vi "Is palindrome-number.vi"(8 "error in (no error)":errorcluster, 11 "x":u64) -> (0 "error out":errorcluster, 3 "T = x is a palindrome":bool)   [LabVIEW 2021, in "Numeric Utilities.lvlib"]
uses:
  Numeric Utilities.lvlib
panel:
  out "x (string representation)":string
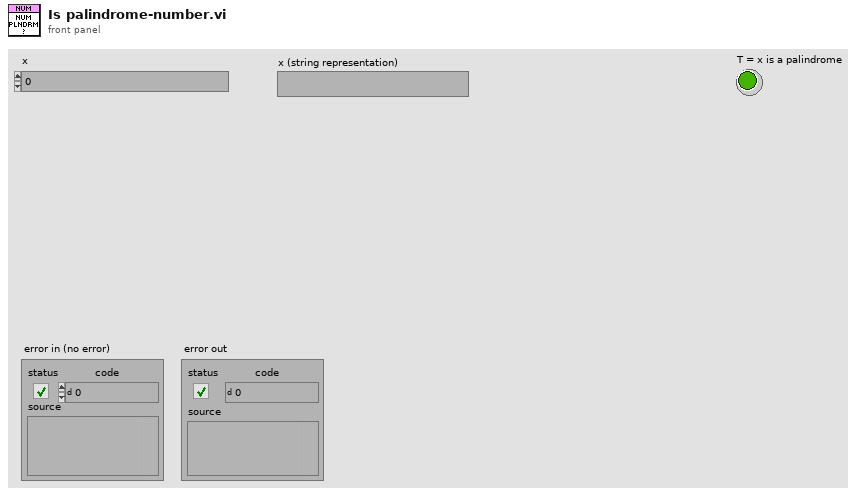
[diagram p1: front panel]
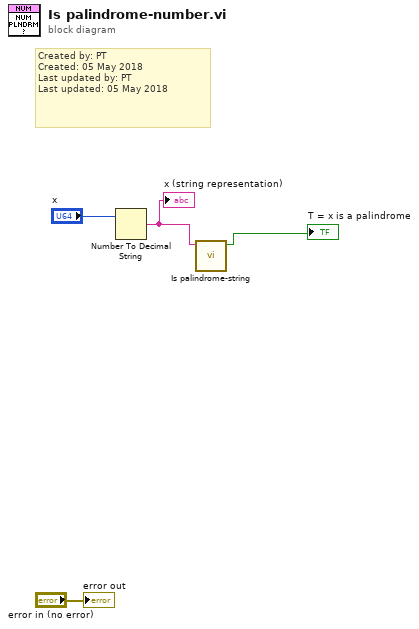
[diagram p0: block diagram]
diagram:
  # "Created by: PT\nCreated: 05 May 2018\nLast updated by: PT\nLast updated: 05 May 2018"
  n1 = Number To Decimal String(number="x") -> (decimal integer string=w2:string)  [unwired: 1 in]
  "x (string representation)" <- w2
  n2 = call "Is palindrome-string.vi"("string in"=w2) -> ("T = string is a palindrome"=→"T = x is a palindrome":bool)  [unwired: 9 in, 1 out]
  "error out" <- "error in (no error)"
